vi "Init with TCP.vi"(8 "error in (no error)":errorcluster, 11 "TCP Connection":refnum<k5>) -> (0 "error out":errorcluster, 3 "Websocket Client out":refnum<class "Websocket Client.lvclass">)   [LabVIEW 2020, in "Stream-Websocket.lvlib" / "Websocket Client.lvclass"]
uses:
  Websocket Client.lvclass
  Websocket Client.lvclass/Websocket Client.ctl
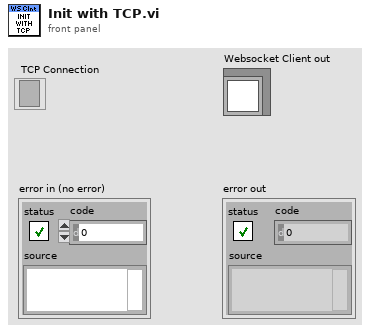
[diagram p1: front panel]
types:
  T1 = typedef "Stream-Websocket.lvlib/Websocket Client.lvclass/Ref Data.ctl" = cluster{"TCP Connection":refnum<k5>, "WS Stream":refnum<class "WebsocketStream.lvclass">, "Connection Loop":refnum<vi>, "Timeout ms":i32, "Server Connection":bool}
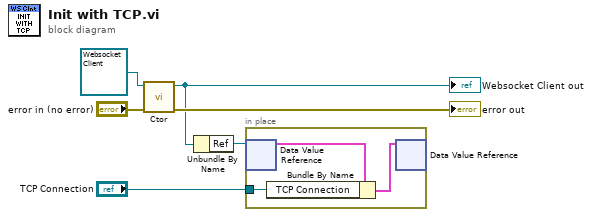
[diagram p0: block diagram]
diagram:
  n1 = call-dynamic "Ctor.vi"("error in (no error)"="error in (no error)", "Websocket Client in"=refnum<class "Websocket Client.lvclass"> refnum) -> ("error out"=→"error out":errorcluster, "Websocket Client out"=w2:refnum<class "Websocket Client.lvclass">)  [unwired: 8 in]
  "Websocket Client out" <- w2
  n2 = Unbundle By Name(w2) -> ("Ref"=w3:refnum<data-value>)
  n3 = in-place {
    in-place-border: "TCP Connection" -> [w7]
    n4 = in-place-dvr #1(w3) -> (w9:T1)  [unwired: 1 out]
    n5 = Bundle By Name(cluster=w9, "TCP Connection"=w7) -> (w8:T1)
    n6 = in-place-dvr #1(w8) -> ()  [unwired: 2 out]
  }
